vi "字符串显示方式.vi"() -> ()   [LabVIEW 2013]
panel:
  in  "十六进制显示":string="Hello World! \nHello World! "
  in  "密码显示":string="Hello World! "
  in  "\\代码显示":string="Hello World! "
  in  "正常显示":string="Hello World! \nHello World! "
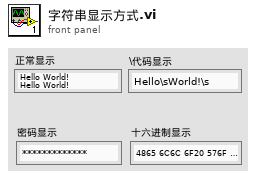
[diagram p1: front panel]
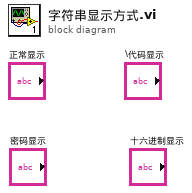
[diagram p0: block diagram]
diagram:
